vi "GetControlSpecificLocalizedPhrase.vi"(7 "Dictionary":T2, 8 "error in (no error)":errorcluster, 9 "Font Info":T1, 10 "Target Language":string, 11 "Control Reference":refnum<vi>) -> (0 "error out":errorcluster, 3 "Control ref out":refnum<vi>)   [LabVIEW 2017, in "JKI Simple Localization.lvlib"]
uses:
  API/JKI Simple Localization.lvlib
  Definitions/Dictionary--Cluster.ctl
  Definitions/Private/Font -- Cluster.ctl
  Definitions/Private/Phrase Dictionary Entry -- Cluster.ctl
  Definitions/Private/Font Info -- Cluster.ctl
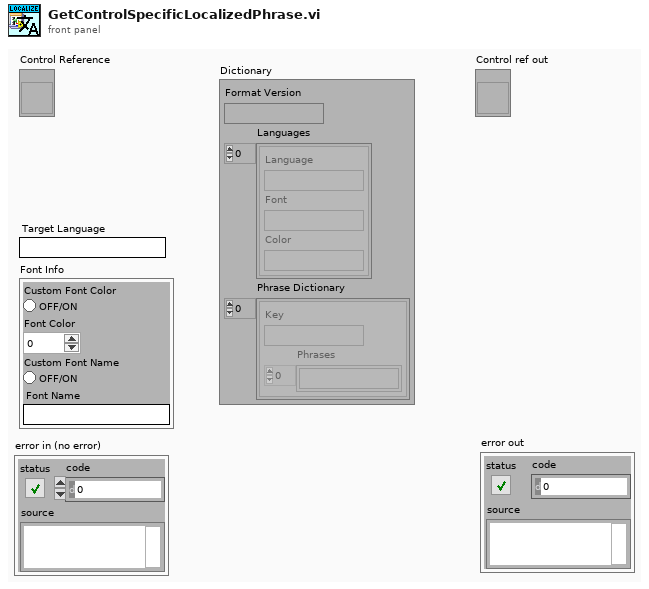
[diagram p1: front panel]
types:
  T1 = typedef "JKI Simple Localization.lvlib/Font Info -- Cluster.ctl" = cluster{"Custom Font Color":bool, "Font Color":u32, "Custom Font Name":bool, "Font Name":string}
  T2 = typedef "JKI Simple Localization.lvlib/Dictionary--Cluster.ctl" = cluster{"Format Version":string, "Languages":T3[], "Phrase Dictionary":T4[]}
  T3 = typedef "JKI Simple Localization.lvlib/Font -- Cluster.ctl" = cluster{"Language":string, "Font":string, "Color":string}
  T4 = typedef "JKI Simple Localization.lvlib/Phrase Dictionary Entry -- Cluster.ctl" = cluster{"Key":string, "Phrases":string[]}
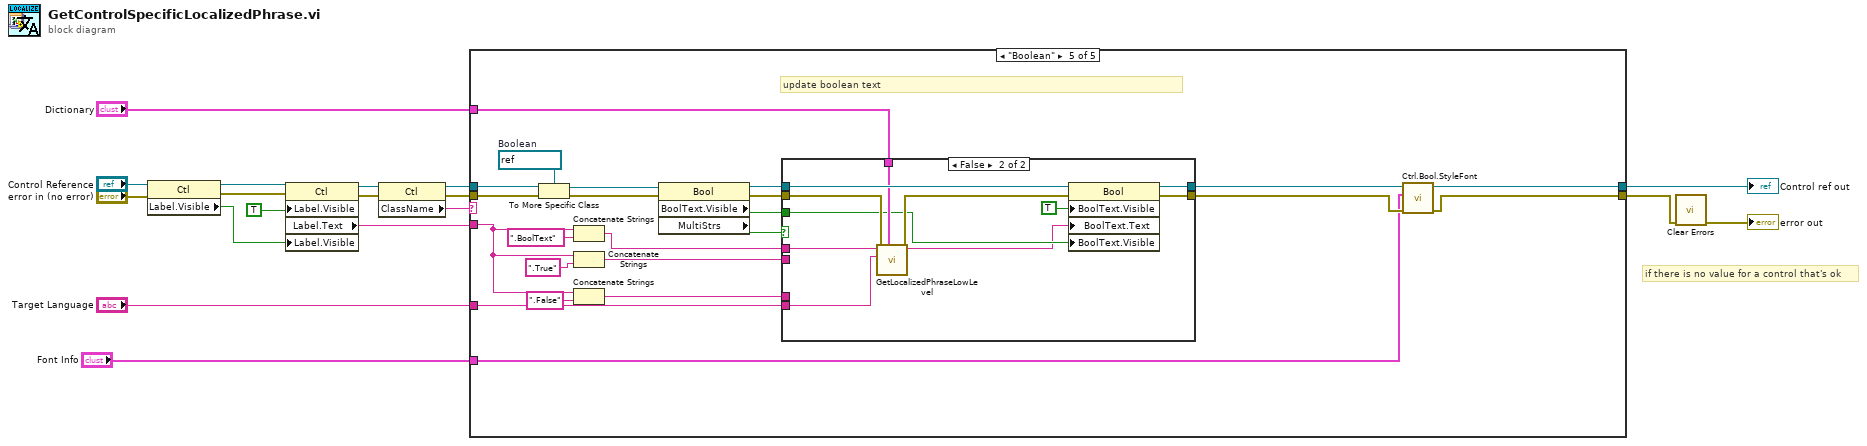
[diagram p0: block diagram]
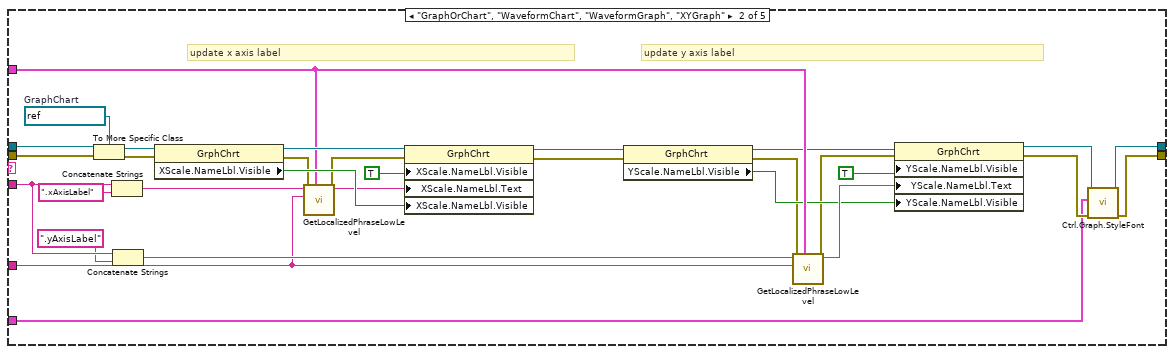
[diagram p3: hidden frame]
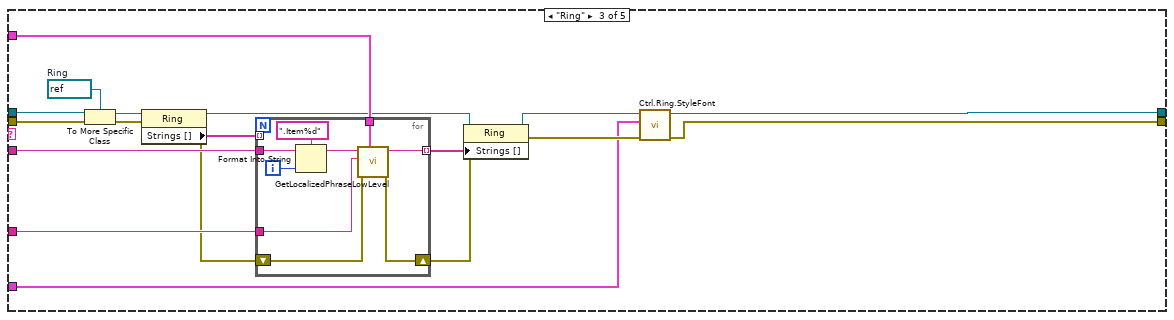
[diagram p4: hidden frame]
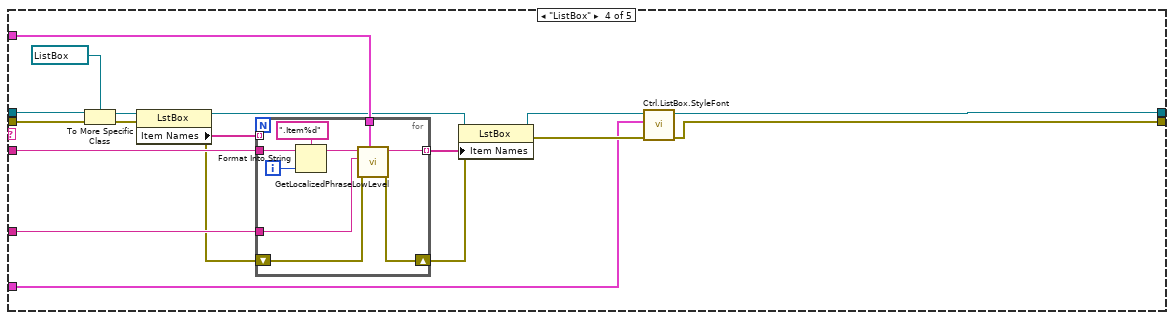
[diagram p5: hidden frame]
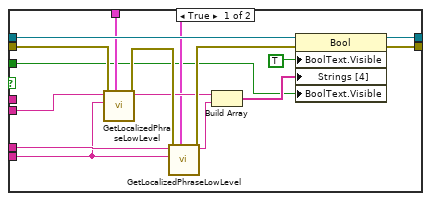
[diagram p6: hidden frame]
diagram:
  # "if there is no value for a control that's ok"
  n1 = property on="Property Node" class="Ctl"(reference="Control Reference", error in="error in (no error)") -> (reference out=w17:refnum<vi>, error out=w14:errorcluster, "Label.Visible"=w16:bool)
  n2 = property on="Property Node" class="Ctl"(reference=w17, error in=w14, "Label.Visible"=TRUE, "Label.Visible"=w16) -> (reference out=w12:refnum<vi>, error out=w8:errorcluster, "Label.Text"=w11:string)
  n3 = property on="Property Node" class="Ctl"(reference=w12, error in=w8) -> (reference out=w10:refnum<vi>, error out=w7:errorcluster, "ClassName"=w18:string)
  n4 = case shown="\"Boolean\"" w18 {
    tunnel: w11 -> [_ w42 w63 w91 w108]
    tunnel: w10 -> [w20 w50 w68 w96 w128]
    tunnel: "Dictionary" -> [_ w39 w62 w90 w119]
    tunnel: "Target Language" -> [_ w28 w61 w89 w116]
    tunnel: w7 -> [w19 w34 w67 w95 w122]
    tunnel: [w20 w25 w55 w81 w114] -> w6
    tunnel: [w19 w23 w53 w82 w112] -> w3
    tunnel: "Font Info" -> [_ w22 w52 w79 w111]
    frame "0", Default {
    }
    frame "GraphOrChart", "WaveformChart", "WaveformGraph", "XYGraph" {
      w48 = refnum<vi> refnum  # GraphChart
      # "update y axis label"
      # "update x axis label"
      n5 = To More Specific Class(target class=w48, reference=w50, error in=w34) -> (specific class reference=w49:refnum<vi>, error out=w33:errorcluster)
      n6 = Concatenate Strings(w42, ".xAxisLabel" ("string")) -> (w46:string)
      n7 = Concatenate Strings(w42, ".yAxisLabel" ("string")) -> (w40:string)
      n8 = property class="GrphChrt"(reference=w49, error in=w33) -> (reference out=w43:refnum<vi>, error out=w32:errorcluster, "XScale.NameLbl.Visible"=w47:bool)
      n9 = call "GetLocalizedPhraseLowLevel.vi"("Dictionary"=w39, "error in (no error)"=w32, "Target Language"=w28, "Key"=w46) -> ("error out"=w31:errorcluster, "Localized Phrase"=w45:string)  [unwired: 6 in]
      n10 = property class="GrphChrt"(reference=w43, error in=w31, "XScale.NameLbl.Visible"=TRUE ("X Scale.Name Label.Visible"), "XScale.NameLbl.Text"=w45, "XScale.NameLbl.Visible"=w47) -> (reference out=w27:refnum<vi>, error out=w21:errorcluster)
      n11 = property class="GrphChrt"(reference=w27, error in=w21) -> (reference out=w38:refnum<vi>, error out=w30:errorcluster, "YScale.NameLbl.Visible"=w35:bool)
      n12 = call "GetLocalizedPhraseLowLevel.vi"("Dictionary"=w39, "error in (no error)"=w30, "Target Language"=w28, "Key"=w40) -> ("error out"=w29:errorcluster, "Localized Phrase"=w36:string)  [unwired: 6 in]
      n13 = property class="GrphChrt"(reference=w38, error in=w29, "YScale.NameLbl.Visible"=TRUE ("X Scale.Name Label.Visible"), "YScale.NameLbl.Text"=w36, "YScale.NameLbl.Visible"=w35) -> (reference out=w26:refnum<vi>, error out=w24:errorcluster)
      n14 = call "Ctrl.Graph.StyleFont.vi"("error in (no error)"=w24, "Font Info"=w22, "Graph Ctrl Ref in"=w26) -> ("error out"=w23:errorcluster, "Graph Ctrl Ref out"=w25:refnum<vi>)  [unwired: 7 in]
    }
    frame "Ring" {
      w69 = refnum<vi> refnum  # Ring
      n15 = To More Specific Class(target class=w69, reference=w68, error in=w67) -> (specific class reference=w66:refnum<vi>, error out=w65:errorcluster)
      n16 = property class="Ring"(reference=w66, error in=w65) -> (reference out=w59:refnum<vi>, error out=w58:errorcluster, "Strings []"=w64:string[])
      n17 = for {
        tunnel: w64 -> [_] mode=indexing
        tunnel: w63 -> [w78]
        tunnel: w62 -> [w75]
        shift-right: [w74] -> w57
        shift-left: w58 -> [w71]
        tunnel: w61 -> [w70]
        tunnel: [w72] -> w60 mode=indexing
        i -> [w76]
        n18 = Format Into String(format string=".Item%d", initial string=w78, w76) -> (resulting string=w73:string)  [unwired: 1 in, 1 out]
        n19 = call "GetLocalizedPhraseLowLevel.vi"("Dictionary"=w75, "error in (no error)"=w71, "Target Language"=w70, "Key"=w73) -> ("error out"=w74:errorcluster, "Localized Phrase"=w72:string)  [unwired: 6 in]
      }
      n20 = property class="Ring"(reference=w59, error in=w57, "Strings []"=w60) -> (reference out=w56:refnum<vi>, error out=w54:errorcluster)
      n21 = call "Ctrl.Ring.StyleFont.vi"("error in (no error)"=w54, "Font Info"=w52, "Ring Ref in"=w56) -> ("error out"=w53:errorcluster, "Ring Ref out"=w55:refnum<vi>)  [unwired: 7 in]
    }
    frame "ListBox" {
      n22 = To More Specific Class(target class=refnum<vi> refnum ("reference out"), reference=w96, error in=w95) -> (specific class reference=w94:refnum<vi>, error out=w93:errorcluster)
      n23 = property class="LstBox"(reference=w94, error in=w93) -> (reference out=w87:refnum<vi>, error out=w86:errorcluster, "Item Names"=w92:string[])
      n24 = for {
        tunnel: w92 -> [_] mode=indexing
        tunnel: w91 -> [w105]
        tunnel: w90 -> [w102]
        shift-right: [w101] -> w85
        shift-left: w86 -> [w98]
        tunnel: w89 -> [w97]
        tunnel: [w99] -> w88 mode=indexing
        i -> [w103]
        n25 = Format Into String(format string=".Item%d", initial string=w105, w103) -> (resulting string=w100:string)  [unwired: 1 in, 1 out]
        n26 = call "GetLocalizedPhraseLowLevel.vi"("Dictionary"=w102, "error in (no error)"=w98, "Target Language"=w97, "Key"=w100) -> ("error out"=w101:errorcluster, "Localized Phrase"=w99:string)  [unwired: 6 in]
      }
      n27 = property class="LstBox"(reference=w87, error in=w85, "Item Names"=w88) -> (reference out=w80:refnum<vi>, error out=w83:errorcluster)
      n28 = call "Ctrl.ListBox.StyleFont.vi"("error in (no error)"=w83, "Font Info"=w79, "Listbox Ref"=w80) -> ("error out"=w82:errorcluster, "Listbox Ref out"=w81:refnum<vi>)  [unwired: 7 in]
    }
    frame "Boolean" {
      w126 = refnum<vi> refnum  # Boolean
      # "update boolean text"
      n29 = To More Specific Class(target class=w126, reference=w128, error in=w122) -> (specific class reference=w127:refnum<vi>, error out=w121:errorcluster)
      n30 = Concatenate Strings(w108, ".BoolText" ("string")) -> (w106:string)
      n31 = Concatenate Strings(w108, ".True" ("string")) -> (w125:string)
      n32 = Concatenate Strings(w108, ".False" ("string")) -> (w123:string)
      n33 = property class="Bool"(reference=w127, error in=w121) -> (reference out=w124:refnum<vi>, error out=w120:errorcluster, "BoolText.Visible"=w118:bool, "MultiStrs"=w117:bool)
      n34 = case shown="False" w117 {
        tunnel: w125 -> [w143 _]
        tunnel: w124 -> [w142 w154]
        tunnel: w123 -> [w141 _]
        tunnel: w116 -> [w129 w144]
        tunnel: w120 -> [w140 w153]
        tunnel: w119 -> [w135 w151]
        tunnel: w118 -> [w132 w149]
        tunnel: w106 -> [_ w148]
        tunnel: [w131 w146] -> w115
        tunnel: [w130 w145] -> w113
        frame True {
          n35 = call "GetLocalizedPhraseLowLevel.vi"("Dictionary"=w135, "error in (no error)"=w140, "Target Language"=w129, "Key"=w143) -> ("error out"=w139:errorcluster, "Localized Phrase"=w137:string)  [unwired: 6 in]
          n36 = call "GetLocalizedPhraseLowLevel.vi"("Dictionary"=w135, "error in (no error)"=w139, "Target Language"=w129, "Key"=w141) -> ("error out"=w138:errorcluster, "Localized Phrase"=w136:string)  [unwired: 6 in]
          n37 = Build Array(w137, w136) -> (w134:string[])
          n38 = property class="Bool"(reference=w142, error in=w138, "BoolText.Visible"=TRUE ("X Scale.Name Label.Visible"), "Strings [4]"=w134, "BoolText.Visible"=w132) -> (reference out=w131:refnum<vi>, error out=w130:errorcluster)
        }
        frame False {
          n39 = call "GetLocalizedPhraseLowLevel.vi"("Dictionary"=w151, "error in (no error)"=w153, "Target Language"=w144, "Key"=w148) -> ("error out"=w152:errorcluster, "Localized Phrase"=w147:string)  [unwired: 6 in]
          n40 = property class="Bool"(reference=w154, error in=w152, "BoolText.Visible"=TRUE ("X Scale.Name Label.Visible"), "BoolText.Text"=w147, "BoolText.Visible"=w149) -> (reference out=w146:refnum<vi>, error out=w145:errorcluster)
        }
      }
      n41 = call "Ctrl.Bool.StyleFont.vi"("error in (no error)"=w113, "Font Info"=w111, "Bool Ref in"=w115) -> ("error out"=w112:errorcluster, "Bool Ref out"=w114:refnum<vi>)  [unwired: 7 in]
    }
  }
  "Control ref out" <- w6
  n42 = call <vilib>:"Clear Errors.vi"("error in (no error)"=w3) -> ("error out"=→"error out":errorcluster)  [unwired: 5 in, 1 out]
